vi "Sine Wave (CDB).vi"(8 "phase":dbl, 9 "frequency":dbl=0.0009765625, 10 "amplitude":dbl=1.0, 11 "samples":i32=1024) -> (3 "complex tone":cdb[](array[numeric]))   [LabVIEW 2013, in "rf-utils.lvlib"]
uses:
  <userlib>/_RF Utils/rf-utils.lvlib
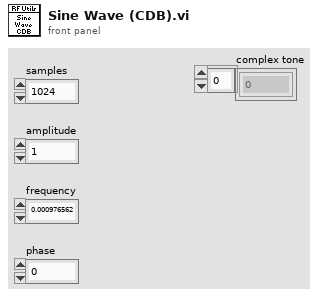
[diagram p1: front panel]
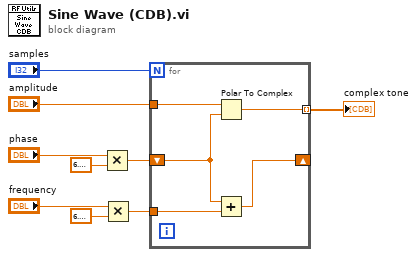
[diagram p0: block diagram]
diagram:
  n1 = Multiply(x="phase", y=6.283185307179586) -> (x*y=w3:dbl)
  n2 = Multiply(x="frequency", y=6.283185307179586) -> (x*y=w2:dbl)
  n3 = for {
    N: "samples" -> [_]
    shift-right: [w11] -> _
    shift-left: w3 -> [w12]
    tunnel: "amplitude" -> [w14]
    tunnel: w2 -> [w13]
    tunnel: [w10] -> w1 mode=indexing
    n4 = Polar To Complex(1:w12, 2:w14) -> (0:w10:cdb)
    n5 = Add(x=w12, y=w13) -> (x+y=w11:dbl)
  }
  "complex tone" <- w1
